vi "ShutdownCurrentMeters.vi"(8 "Error In":errorcluster, 10 "Number of 6485s":i32, 11 "Current Meters In":refnum<visa-resource-name>[](array[refnum])) -> (0 "Error Out":errorcluster, 3 "Current Meters Out":refnum<visa-resource-name>[](array[refnum]))   [LabVIEW 2012]
uses:
  libs/Keithley-6485/Keithley-6485.lvlib
  libs/Keithley-6482/Keithley-6482.lvlib
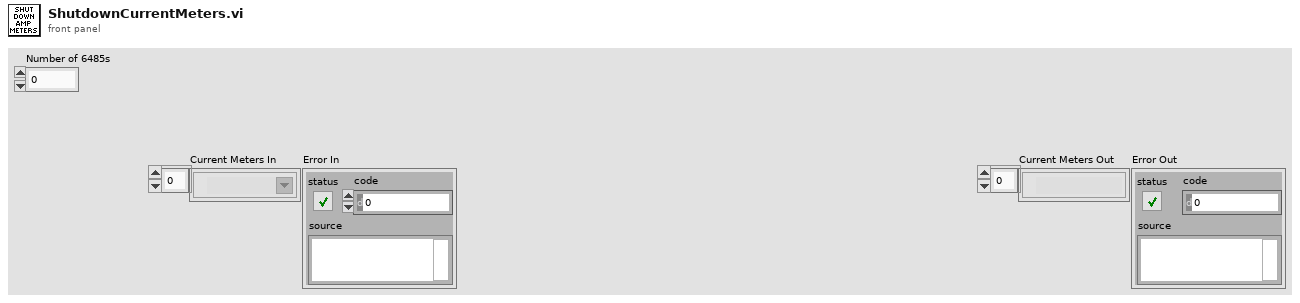
[diagram p1: front panel]
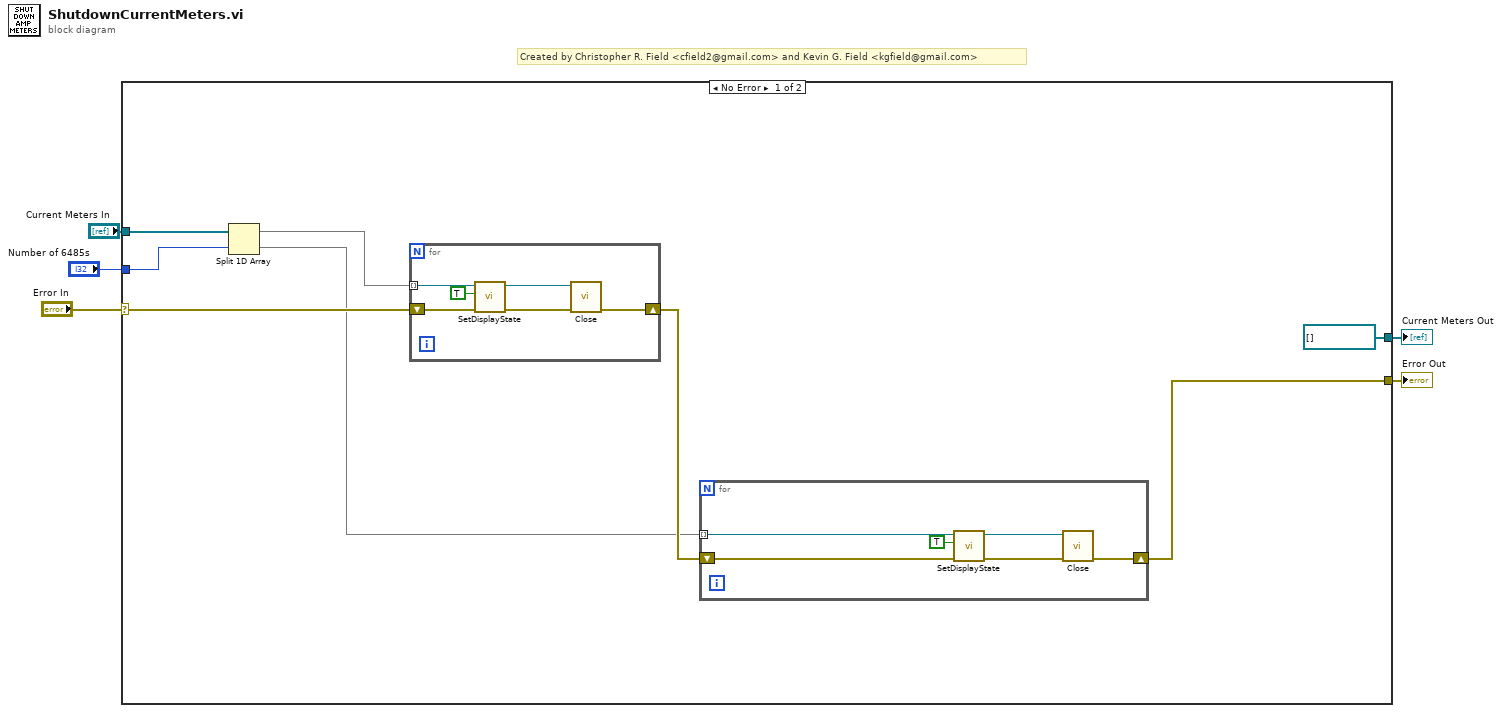
[diagram p0: block diagram]
diagram:
  # "Created by Christopher R. Field <cfield2@gmail.com> and Kevin G. Field <kgfield@gmail.com>"
  n1 = case shown="No Error" "Error In" {
    selector: "Error In" -> [w12 w26]
    tunnel: "Current Meters In" -> [w9 w27]
    tunnel: [refnum<visa-resource-name>[] [] w27] -> w4
    tunnel: [w10 w26] -> w3
    tunnel: "Number of 6485s" -> [w8 _]
    frame No Error {
      n2 = Split 1D Array(array=w9, index=w8) -> (first subarray=w7:refnum<visa-resource-name>[], second subarray=w6:refnum<visa-resource-name>[])
      n3 = for {
        tunnel: w7 -> [w25] mode=indexing
        shift-right: [w21] -> w11
        shift-left: w12 -> [w20]
        n4 = call "SetDisplayState.vi"("Error In"=w20, "Enabled?"=TRUE, "Keithley 6485 In"=w25) -> ("Error Out"=w23:errorcluster, "Keithley 6485 Out"=w24:refnum<visa-resource-name>)  [unwired: 7 in]
        n5 = call "Close.vi"("Error In"=w23, "Keithley 6485 In"=w24) -> ("Error Out"=w21:errorcluster)  [unwired: 9 in]
      }
      n6 = for {
        shift-right: [w16] -> w10
        shift-left: w11 -> [w15]
        tunnel: w6 -> [w14] mode=indexing
        n7 = call "SetDisplayState.vi"("Error In"=w15, "Enabled?"=TRUE, "Keithley 6482 In"=w14) -> ("Error Out"=w18:errorcluster, "Keithley 6482 Out"=w19:refnum<visa-resource-name>)  [unwired: 7 in]
        n8 = call "Close.vi"("Error In"=w18, "Keithley 6482 In"=w19) -> ("Error Out"=w16:errorcluster)  [unwired: 9 in]
      }
    }
    frame Error {
    }
  }
  "Current Meters Out" <- w4
  "Error Out" <- w3
